vi "Find all property nodes for a cluster.vi"() -> ()   [LabVIEW 2010]
uses:
  <vilib>/Utility/traverseref.llb/VI Scripting - Traverse.lvlib
  <vilib>/Utility/traverseref.llb/TRef TravTarget.ctl
panel:
  out "Property Nodes":refnum<vi>[](array[refnum])
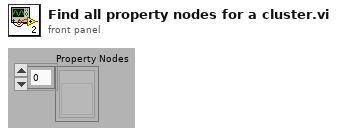
[diagram p1: front panel]
types:
  T1 = typedef "TRef TravTarget.ctl" = enum16{"FP", "BD", "Other"}
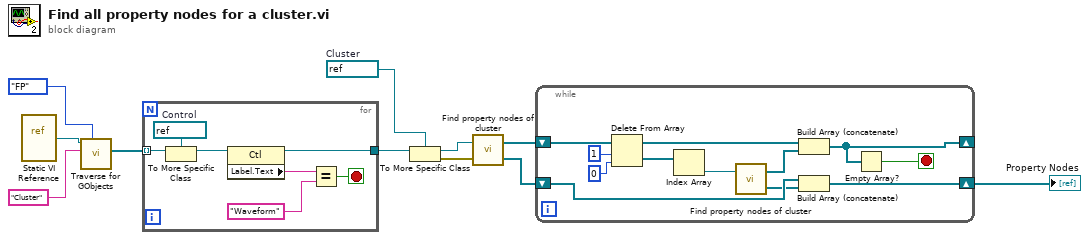
[diagram p0: block diagram]
diagram:
  w7 = refnum<vi> refnum  # Cluster
  n1 = vi-ref "Static VI Reference"() -> ("vi reference"=w1:refnum<vi>)
  n2 = call <vilib>:"Traverse for GObjects.vi"("Traverse Target"=TRef_TravTarget."FP", "Class Name"="Cluster", "VI Refnum"=w1) -> ("References"=w9:refnum<vi>[])  [unwired: 5 in, 3 out]
  n3 = for {
    tunnel: w9 -> [w18] mode=indexing
    tunnel: [w13] -> w8
    stop <- w15 stop-if-true
    w12 = refnum<vi> refnum  # Control
    n4 = To More Specific Class(target class=w12, reference=w18) -> (specific class reference=w17:refnum<vi>)  [unwired: 1 in, 1 out]
    n5 = property class="Ctl"(reference=w17) -> (reference out=w13:refnum<vi>, "Label.Text"=w16:string)  [unwired: 1 in, 1 out]
    n6 = Equal?(x=w16, y="Waveform") -> (x = y?=w15:bool)
  }
  n7 = To More Specific Class(target class=w7, reference=w8) -> (specific class reference=w6:refnum<vi>, error out=w5:errorcluster)  [unwired: 1 in]
  n8 = call "Find property nodes of cluster.vi"("error in"=w5, "Clust Refnum"=w6) -> ("Property Nodes"=w3:refnum<vi>[], "Array of refs to embedded clusters"=w4:refnum<vi>[])
  n9 = while {
    shift-right: [w23] -> _
    shift-left: w4 -> [w30]
    shift-right: [w20] -> w2
    shift-left: w3 -> [w22]
    stop <- w19 stop-if-true
    n10 = Delete From Array(array=w30, length=1, index=0) -> (deleted portion=w27:refnum<vi>[], array with subset deleted=w24:refnum<vi>[])
    n11 = Index Array(array=w27) -> (element=w26:refnum<vi>)  [unwired: 1 in]
    n12 = call "Find property nodes of cluster.vi"("Clust Refnum"=w26) -> ("Property Nodes"=w21:refnum<vi>[], "Array of refs to embedded clusters"=w25:refnum<vi>[])  [unwired: 1 in]
    n13 = Build Array (concatenate)(w24, w25) -> (w23:refnum<vi>[])
    n14 = Build Array (concatenate)(w22, w21) -> (w20:refnum<vi>[])
    n15 = Empty Array?(array=w23) -> (empty?=w19:bool)
  }
  "Property Nodes" <- w2
